vi "RSZVB Get Time Domain Start Time.vi"(8 "error in (no error)":errorcluster {"code" format="%.0x"}, 10 "Channel (Trace) (1)":i32=1, 11 "VISA session":refnum<visa-resource-name>) -> (0 "error out":errorcluster {"code" format="%.0x"}, 2 "Start Time":dbl format="%^.3e", 3 "dup VISA session":refnum<visa-resource-name>)   [LabVIEW 2011]
doc: "This VI queries the start time of the diagram in time domain.\n\nRemote-control command(s):\nCALCulate<Ch/Tr>:TRANsform:TIME:STARt?"
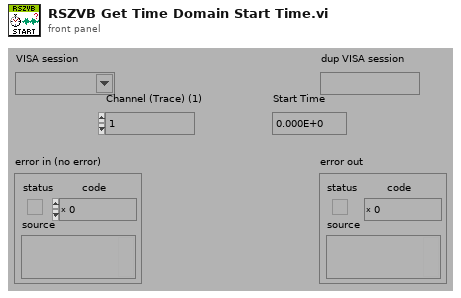
[diagram p1: front panel]
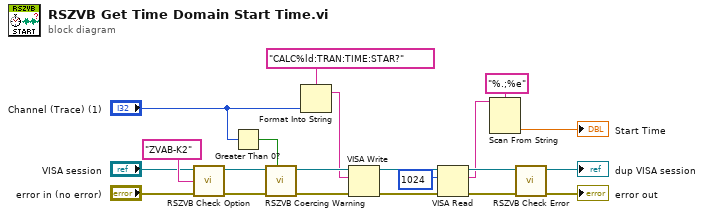
[diagram p0: block diagram]
diagram:
  n1 = call "RSZVB Check Option.vi"("error in (no error)"="error in (no error)", "Options"="ZVAB-K2", "VISA session"="VISA session") -> ("error out"=w5:errorcluster, "dup VISA session"=w6:refnum<visa-resource-name>)  [unwired: 7 in]
  n2 = Greater Than 0?(x="Channel (Trace) (1)") -> (x > 0?=w2:bool)
  n3 = call "RSZVB Coercing Warning.vi"("In Range?"=w2, "error in (no error)"=w5, "VISA session"=w6) -> ("error out"=w19:errorcluster, "dup VISA session"=w20:refnum<visa-resource-name>)  [unwired: 7 in]
  n4 = Format Into String(format string="CALC%ld:TRAN:TIME:STAR?", "Channel (Trace) (1)") -> (resulting string=w18:string)  [unwired: 2 in, 1 out]
  n5 = VISA Write(VISA resource name=w20, write buffer=w18, error in (no error)=w19) -> (VISA resource name out=w15:refnum<visa-resource-name>, error out=w17:errorcluster)  [unwired: 1 out]
  n6 = VISA Read(VISA resource name=w15, byte count=u32 1024 ("byte count (0)"), error in (no error)=w17) -> (VISA resource name out=w14:refnum<visa-resource-name>, read buffer=w11:string, error out=w13:errorcluster)  [unwired: 1 out]
  n7 = Scan From String(format string="%.;%e", input string=w11) -> (output 1=→"Start Time":dbl)  [unwired: 3 in, 3 out]
  n8 = call "RSZVB Check Error.vi"("error in (no error)"=w13, "VISA session"=w14) -> ("error out"=→"error out":errorcluster, "dup VISA session"=→"dup VISA session":refnum<visa-resource-name>)  [unwired: 8 in]
